vi "get_general_location.vi"(8 "error in (no error)":errorcluster, 11 "Mission in":refnum<class "Mission.lvclass">) -> (0 "error out":errorcluster, 2 "General Location":T1 {"North" format="%#_10f"; "East" format="%#_8f"}, 3 "Mission out":refnum<class "Mission.lvclass">)   [LabVIEW 2011, in "Mission.lvclass"]
doc: "Returns a general location of the mission, usable for other missions that want to send the boat in the right general direction."
uses:
  Mission.lvclass
  2 Typedefs/UTM Location.ctl
  Mission.lvclass/Mission.ctl
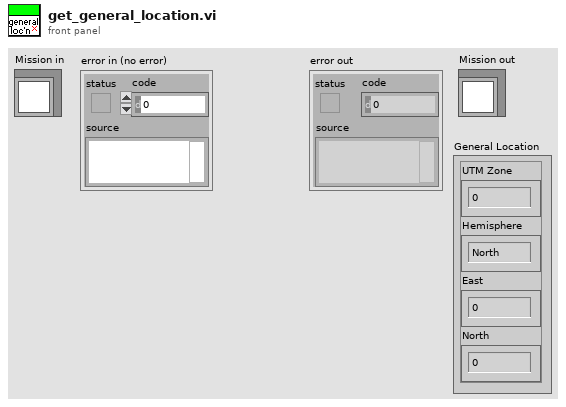
[diagram p1: front panel]
types:
  T1 = typedef "UTM Location.ctl" = cluster{"UTM Zone":dbl, "Hemisphere":enum16{"North", "South"}, "East":dbl, "North":dbl}
  T2 = enum16{"Round Buoy", "Drive", "Pass Buoys", "Station Keeping"}
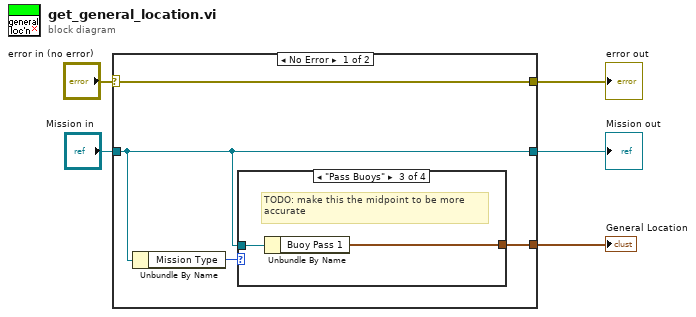
[diagram p0: block diagram]
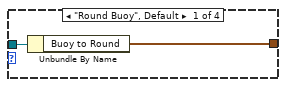
[diagram p2: hidden frame]
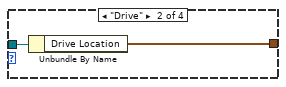
[diagram p3: hidden frame]
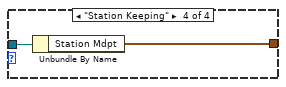
[diagram p4: hidden frame]
diagram:
  n1 = case shown="No Error" "error in (no error)" {
    selector: "error in (no error)" -> [w9 w19]
    tunnel: [w9 w19] -> w4
    tunnel: [w7 w18] -> w2
    tunnel: "Mission in" -> [w7 w18]
    tunnel: [w6 _] -> w1
    frame No Error {
      n2 = Unbundle By Name(w7) -> ("Mission Type"=w8:T2)
      n3 = case shown="\"Pass Buoys\"" w8 {
        tunnel: w7 -> [w11 w13 w15 w16]
        tunnel: [w10 w12 w14 w17] -> w6
        frame "Round Buoy", Default {
          n4 = Unbundle By Name(w11) -> ("Buoy to Round"=w10:T1)
        }
        frame "Drive" {
          n5 = Unbundle By Name(w13) -> ("Drive Location"=w12:T1)
        }
        frame "Pass Buoys" {
          # "TODO: make this the midpoint to be more\naccurate"
          n6 = Unbundle By Name(w15) -> ("Buoy Pass 1"=w14:T1)
        }
        frame "Station Keeping" {
          n7 = Unbundle By Name(w16) -> ("Station Mdpt"=w17:T1)
        }
      }
    }
    frame Error {
    }
  }
  "error out" <- w4
  "Mission out" <- w2
  "General Location" <- w1
